vi "CalculateDummyCaseStructureSize.vi"(8 "Error In":errorcluster, 11 "VI in":refnum<vi>) -> (0 "Error Out":errorcluster, 1 "Dummy case structure size":T1, 2 "Dummy case structure position":T2, 3 "VI ref out (dup)":refnum<vi>)   [LabVIEW 2017, in "ErrorStructureDrawer.lvlib"]
doc: "Calculates the size and position for creating a dummy case structure.\n\nIt is created at the same height as the height of the bounding box of all top-level controls and indicators. It is positioned vertically such that it fits within that control/indicator bounding box. Horizontally, it is positioned in the middle of that bounding box. The reason for doing this is to ensure that the \"real\" case structure (to be used as the error case) will be sufficiently large in the vertical direction to allow all wires between controls/indicators and the code inside the structure to pass through the left or right borders. Otherwise there is a risk of getting the wire tunnels on the top or bottom borders, which doesn't look good."
uses:
  ErrorStructureDrawer.lvlib
  <vilib>/Utility/miscctls.llb/LVPointTypeDef.ctl
  <vilib>/Utility/miscctls.llb/LVBoundsTypeDef.ctl
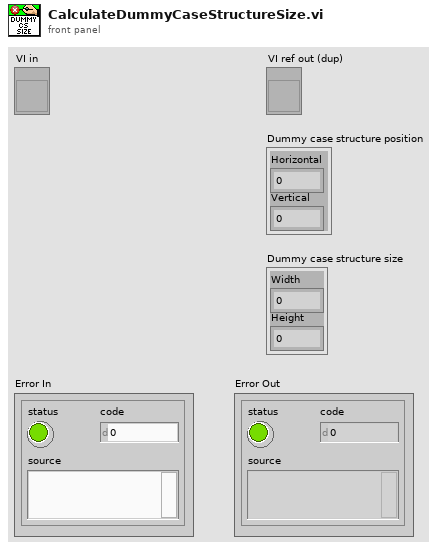
[diagram p1: front panel]
types:
  T1 = typedef "LVBoundsTypeDef.ctl" = cluster{"Width":u32, "Height":u32}
  T2 = typedef "LVPointTypeDef.ctl" = cluster{"Horizontal":i16, "Vertical":i16}
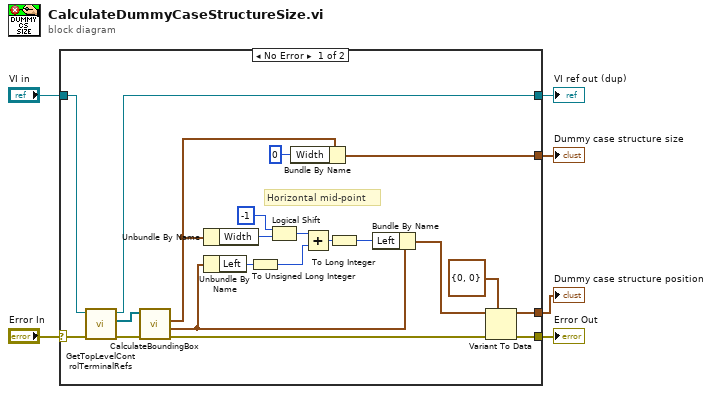
[diagram p0: block diagram]
diagram:
  n1 = case shown="No Error" "Error In" {
    selector: "Error In" -> [w8 w29]
    tunnel: [w22 _] -> w6
    tunnel: "VI in" -> [w18 w28]
    tunnel: [w16 w28] -> w4
    tunnel: [w9 _] -> w3
    tunnel: [w7 w29] -> w1
    frame No Error {
      # "Horizontal mid-point"
      n2 = call "GetTopLevelControlTerminalRefs.vi"("error in (no error)"=w8, "VI ref in"=w18) -> ("error out"=w17:errorcluster, "Control terminals on top-level"=w19:refnum<vi>[], "VI ref out (dup)"=w16:refnum<vi>)  [unwired: 7 in]
      n3 = call "CalculateBoundingBox.vi"("error in (no error)"=w17, "Items"=w19) -> ("error out"=w12:errorcluster, "Current bounding box position"=w15:cluster{"Left":i32, "Top":i32}, "Size of bounding box for items"=w21:T1)  [unwired: 6 in, 1 out]
      n4 = Unbundle By Name(w21) -> ("Width"=w23:u32)
      n5 = Unbundle By Name(w15) -> ("Left"=w26:i32)
      n6 = To Unsigned Long Integer(number=w26) -> (unsigned 32bit integer=w27:u32)
      n7 = Logical Shift(y=i16 -1, x=w23) -> (x << y=w25:u32)
      n8 = Bundle By Name(cluster=w21, "Width"=u32 0) -> (w22:T1)
      n9 = Add(x=w25, y=w27) -> (x+y=w14:u32)
      n10 = To Long Integer(number=w14) -> (32bit integer=w13:i32)
      n11 = Bundle By Name(cluster=w15, "Left"=w13) -> (w11:cluster{"Left":i32, "Top":i32})
      n12 = Variant To Data(error in=w12, type=T2 {"Horizontal"=0, "Vertical"=0} ("location"), Variant=w11) -> (data=w9:T2, error out=w7:errorcluster)
    }
    frame Error {
    }
  }
  "Dummy case structure position" <- w3
  "Dummy case structure size" <- w6
  "VI ref out (dup)" <- w4
  "Error Out" <- w1
